vi "Set Up Dialog - Drop Counter.vi"() -> ()   [LabVIEW 2014]
panel:
  out "Calibration Instructions":string="1. Connect the sensor to your myDAQ as shown in the diagram above.\n\n2. Set the sensor so that drops fall directly through the center of the hole and are about 1 inch above the optical slot. \n\n3. Test your system by sending a few drops through the sensor so you see the signal on the waveform chart. Set the drip rate to 2 seconds per drop or slower.\n\n4. Set the Threshold so that the voltage signal rises above it when a drop is detected but well above the baseline of the signal."
  # "Drop Counter - Set Up"
  # "Drop Counter (DCN - 100)"
  # "iWorx"
  # "Sensor"
  # "DCN - 100"
  # "myDAQ"
  # "Computer"
  # "Adaptor"
  # "Connection Diagram"
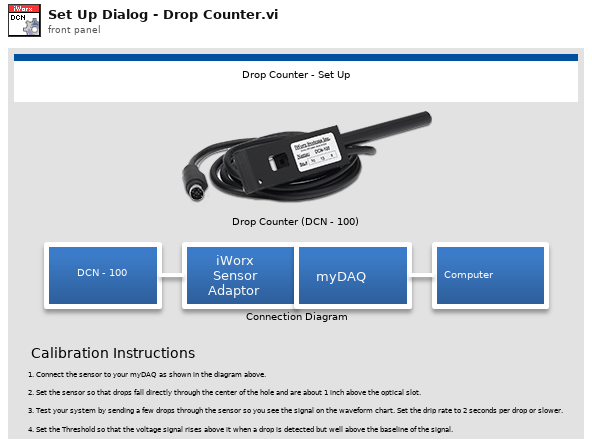
[diagram p1: front panel]
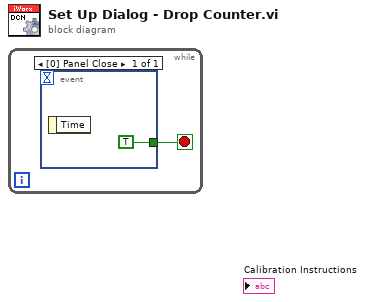
[diagram p0: block diagram]
diagram:
  n1 = while {
    stop <- w1 stop-if-true
    n2 = event shown="[0] Panel Close" {
      selector: _ -> [_]
      dyn-events: _ -> [_]
      timeout: _ -> [_]
      tunnel: [TRUE] -> w1
      event Panel Close {
        n3 = event-data() -> ()  [unwired: 1 in, 1 out]
      }
    }
  }
